vi "Read Error.vi"(8 "error in (no error)":errorcluster, 9 "timeout in ms (0)":i32, 11 "Interface in":refnum<class "Interface.lvclass">) -> (0 "error out":errorcluster, 1 "timed out?":bool, 2 "error":errorcluster, 3 "Interface out":refnum<class "Interface.lvclass">)   [LabVIEW 2017, in "DSF Core.lvlib" / "Interface.lvclass"]
uses:
  Interface.lvclass
  Interface.lvclass/Interface.ctl
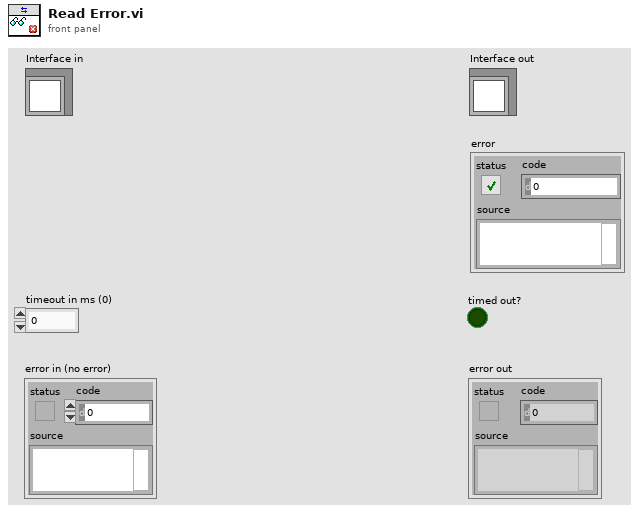
[diagram p1: front panel]
types:
  T1 = typedef "DSF Core.lvlib/FIFO Flags.ctl" = cluster{"Infinite Timeouts":bool}
  T2 = typedef "DSF Core.lvlib/Interface.lvclass/Error Queue Ref.ctl" = refnum<queue>
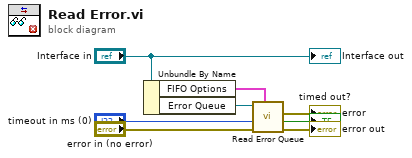
[diagram p0: block diagram]
diagram:
  n1 = Unbundle By Name("Interface in") -> ("FIFO Options"=w2:T1, "Error Queue"=w3:T2)
  n2 = call "Read Error Queue.vi"("FIFO Options"=w2, "error in (no error)"="error in (no error)", "timeout in ms (0)"="timeout in ms (0)", "Error Queue in"=w3) -> ("error out"=→"error out":errorcluster, "timed out?"=→"timed out?":bool, "element"=→"error":errorcluster)  [unwired: 4 in, 1 out]
  "Interface out" <- "Interface in"
